vi "uintSubstract.vi"(8 "Error in (no error)":errorcluster, 10 "Uint2 in":refnum<class "UintClass.lvclass">, 11 "Uint1 in":refnum<class "UintClass.lvclass">) -> (0 "Error out":errorcluster, 1 "Timing":u32, 3 "Uint1 + Uint2":refnum<class "UintClass.lvclass">, 5 "Timeout?":bool)   [LabVIEW 2011, in "UintClass.lvclass"]
uses:
  UintClass.lvclass
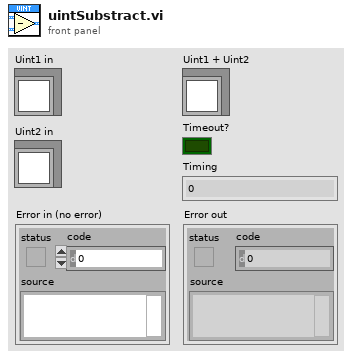
[diagram p1: front panel]
types:
  T1 = typedef "UintClass.lvclass/timeout.ctl" = i32
  T2 = typedef "UintClass.lvclass/enumBase.ctl" = u16
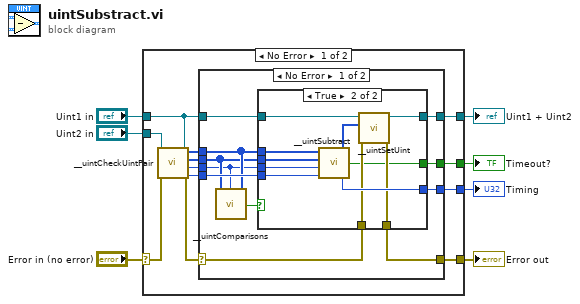
[diagram p0: block diagram]
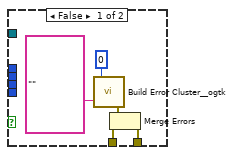
[diagram p2: hidden frame]
diagram:
  n1 = case shown="No Error" "Error in (no error)" {
    selector: "Error in (no error)" -> [w16 w48]
    tunnel: [w14 w48] -> w6
    tunnel: "Uint2 in" -> [w17 _]
    tunnel: "Uint1 in" -> [w9 _]
    tunnel: [w19 _] -> w3
    tunnel: [w18 _] -> w2
    tunnel: [w8 _] -> w1
    frame No Error {
      n2 = call "__uintCheckUintPair.vi"("Error in (no error)"=w16, "Uint2 in"=w17, "Uint1 in"=w9) -> ("Error out"=w15:errorcluster, "Timeout (-1)"=w11:T1, "Uint2 out"=w12:u8[], "Uint1 out"=w13:u8[], "Base out"=w10:T2)  [unwired: 4 in]
      n3 = case shown="No Error" w15 {
        selector: w15 -> [w26 w47]
        tunnel: [w30 _] -> w19
        tunnel: [w29 _] -> w18
        tunnel: [w25 w47] -> w14
        tunnel: w13 -> [w23 _]
        tunnel: w12 -> [w22 _]
        tunnel: w11 -> [w20 _]
        tunnel: w10 -> [w28 _]
        tunnel: w9 -> [w27 _]
        tunnel: [w24 _] -> w8
        frame No Error {
          n4 = call "__uintComparisons.vi"("Timeout (-1)"=w20, "Uint2 in"=w22, "Uint1 in"=w23) -> ("Uint1 >= Uint2"=w21:bool)  [unwired: 1 in, 7 out]
          n5 = case shown="True" w21 {
            tunnel: [_ w46] -> w30
            tunnel: [_ w44] -> w29
            tunnel: w20 -> [_ w43]
            tunnel: w28 -> [_ w42]
            tunnel: w27 -> [_ w41]
            tunnel: w26 -> [w35 w40]
            tunnel: [w34 w39] -> w25
            tunnel: [_ w38] -> w24
            tunnel: w23 -> [_ w37]
            tunnel: w22 -> [_ w36]
            frame False {
              n6 = call <userlib>:"Build Error Cluster__ogtk.vi"("String to Prepend to source (\"\")"="" ("String to Prepend to source (\"\")"), "code"=0) -> ("error out"=w33:errorcluster)
              n7 = Merge Errors(w33, w35) -> (w34:errorcluster)
            }
            frame True {
              n8 = call "__uintSubtract.vi"("Uint1 in"=w37, "Uint2 in"=w36, "Timeout (-1)"=w43, "Base (decimal)"=w42) -> ("Uint1 - Uint2"=w45:u8[], "Timeout?"=w38:bool, "Timing substraction"=w46:u32)  [unwired: 1 in]
              n9 = call "__uintSetUint.vi"("Error in (no error)"=w40, 10:"Uint in"=w45, 11:"Uint in"=w41) -> ("Error out"=w39:errorcluster, "Uint out"=w44:refnum<class "UintClass.lvclass">)  [unwired: 7 in]
            }
          }
        }
        frame Error {
        }
      }
    }
    frame Error {
    }
  }
  "Error out" <- w6
  "Uint1 + Uint2" <- w2
  "Timing" <- w3
  "Timeout?" <- w1
